vi "risingEdge (SubVI).vi"(11 "input":bool) -> (3 "risingTure":bool)   [LabVIEW 2020]
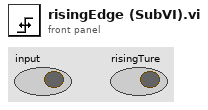
[diagram p1: front panel]
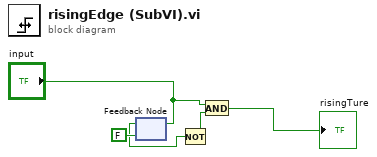
[diagram p0: block diagram]
diagram:
  n1 = feedback #1(FALSE ("B")) -> (w3:bool)
  n2 = feedback-in #1("input") -> ()
  n3 = Not(x=w3) -> (.not. x?=w2:bool)
  n4 = And(x="input", y=w2) -> (x .and. y?=→"risingTure":bool)
